vi "Get PSU Field.vi"(8 "error in (no error)":errorcluster, 11 "Instrument.1820 in":refnum<class "Instrument.Oxford1820.lvclass">) -> (0 "error out":errorcluster, 2 "PSU Field (T)":dbl, 3 "Instrument.1820 in":refnum<class "Instrument.Oxford1820.lvclass">)   [LabVIEW 2019, in "Instrument.Oxford1820.lvclass"]
uses:
  Instrument.Oxford1820.lvclass
  1eda0456-619c-498c-ad55-843362e50380.vi
  Typedefs/Instrument.Oxford1820.protectedCommands-enum.ctl
  C:/Program Files/National Instruments/LabVIEW 2019/user.lib/LevyLab/Instrument Framework/Instrument Types/Cryostat/Instrument.Cryostat.lvclass
  C:/Program Files/National Instruments/LabVIEW 2019/user.lib/LevyLab/Instrument Framework/Instrument/Instrument.lvclass
  C:/Program Files/National Instruments/LabVIEW 2019/vi.lib/JKI/JKI SMO/SMO/SMO.lvclass
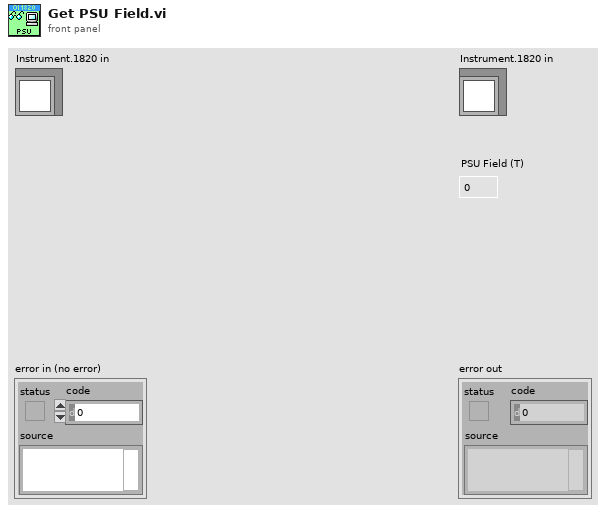
[diagram p1: front panel]
types:
  T1 = typedef "Instrument.Oxford1820.lvclass/Instrument.Oxford1820.protectedCommands-enum.ctl" = enum16{"setAction", "setTarget", "setSwitchHeat", "setLambda", "setFillMode", "setNeedleValve", "getStatus", "getTarget", "getSwitchHeat", "getPSUField", "setSequenceStatus"}
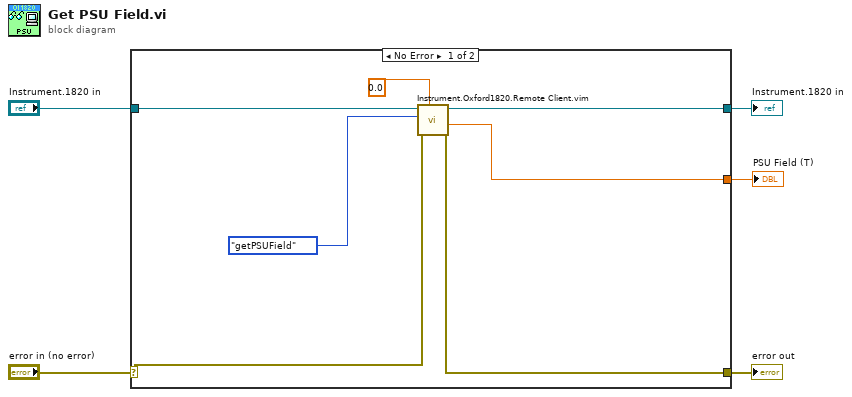
[diagram p0: block diagram]
diagram:
  n1 = case shown="No Error" "error in (no error)" {
    selector: "error in (no error)" -> [w12 w14]
    tunnel: [w7 w14] -> w4
    tunnel: "Instrument.1820 in" -> [w11 w13]
    tunnel: [w8 _] -> w2
    tunnel: [w10 w13] -> w1
    frame No Error {
      n2 = call "Instrument.Oxford1820.Remote Client.vim"("Data Out type"=0.0, "error in (no error)"=w12, "Commands"=Instrument.Oxford1820.protectedCommands-enum."getPSUField", "Instrument.1820 in"=w11) -> ("error out"=w7:errorcluster, "Data out"=w8:dbl, "Instrument.1820 out"=w10:refnum<class "Instrument.Oxford1820.lvclass">)  [unwired: 5 in]
    }
    frame Error {
    }
  }
  "error out" <- w4
  "Instrument.1820 in" <- w1
  "PSU Field (T)" <- w2
